vi "BRig_dataLC_ENL_PreR_Count_l2.vi"() -> (2 "output_ENL_PreR_Count_l2":i32)   [LabVIEW 2014]
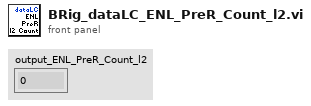
[diagram p1: front panel]
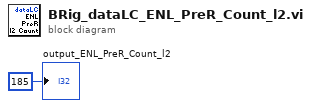
[diagram p0: block diagram]
diagram:
  "output_ENL_PreR_Count_l2" <- 185 ("output_iBlock")
